vi "MeasAction.vi"(8 "error in (no error)":errorcluster caption="entrée d'erreur (pas d'erreur)", 9 "CurvePointIndex":i32, 10 "AllPointIndex":i32, 11 "InstrClassIn":refnum<class "LSCI332.lvclass"> caption="DNL_LabVIEW Object in") -> (0 "error out":errorcluster caption="sortie d'erreur", 2 "MeasDatOut":dbl[](array[numeric]), 3 "InstrClassOut":refnum<class "LSCI332.lvclass"> caption="DNL_LabVIEW Object out")   [LabVIEW 2019, in "LSCI332.lvclass"]
uses:
  LSCI332.lvclass
  C:/Programmes LabView/LabScanV1A/DevicesClass/BaseDevice/BaseDevice.lvclass
  LSCI332.lvclass/LSCI332.ctl
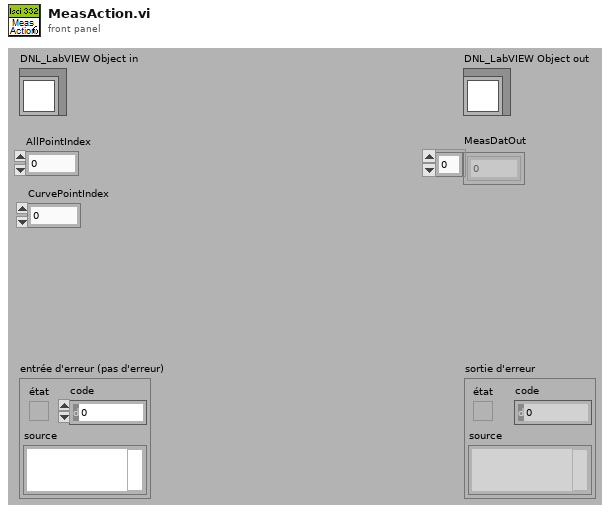
[diagram p1: front panel]
types:
  T1 = typedef "LSCI332.lvclass/LSCI332_Func.ctl" = enum16{"Read_InputA (K,S)", "Read_InputA&Heater (K,S,%,W)", "Read_InputB (K,S)", "Read_InputB&Heater (K,S,%,W)", "Read_Heater (%,W)", "Read_InputA&B(K,S,K,S)", "Read_InputA&B&Heater (K,S,K,S,%,W)", "Scan_Loop1(K,S)", "Scan_Loop2(K,S)"}
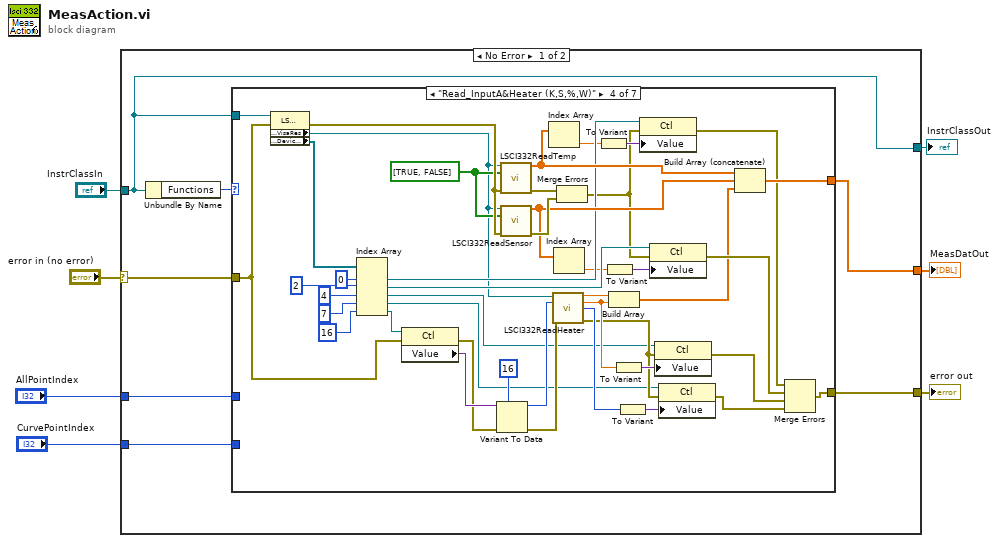
[diagram p0: block diagram]
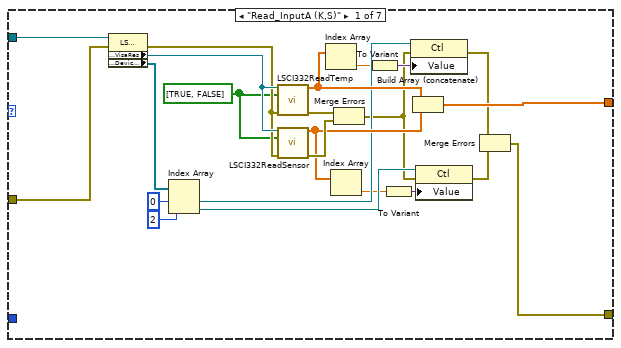
[diagram p2: hidden frame]
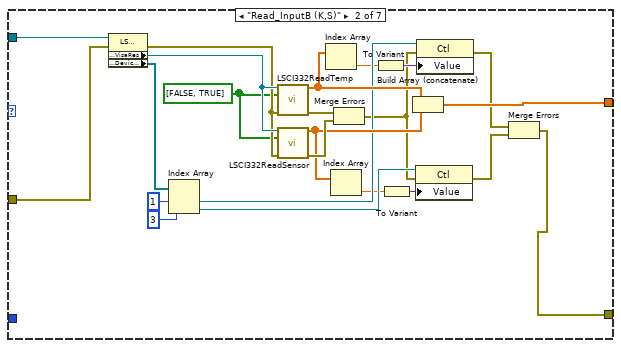
[diagram p3: hidden frame]
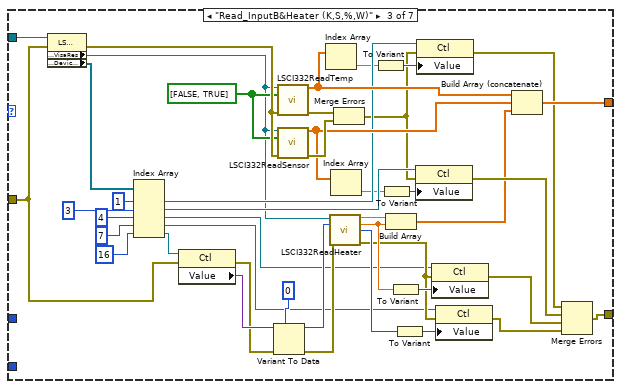
[diagram p4: hidden frame]
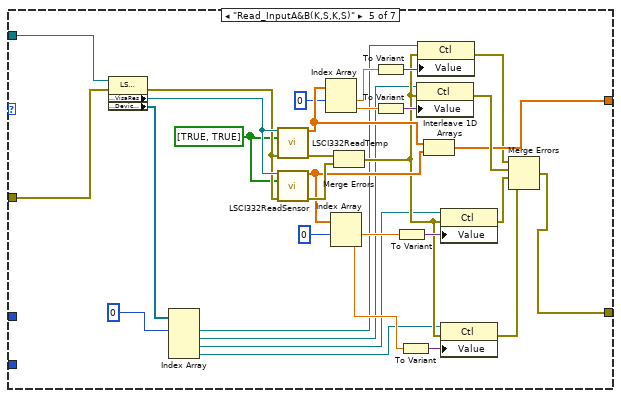
[diagram p5: hidden frame]
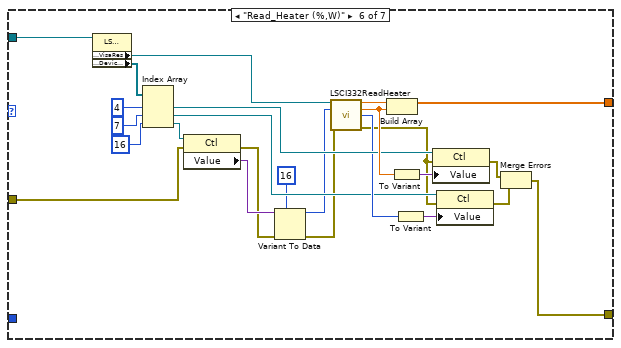
[diagram p6: hidden frame]
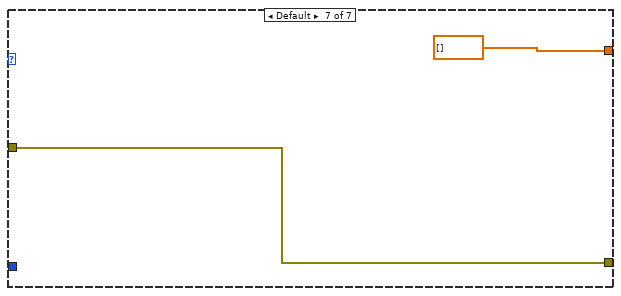
[diagram p7: hidden frame]
diagram:
  n1 = case shown="No Error" "error in (no error)" {
    selector: "error in (no error)" -> [w10 w206]
    tunnel: "InstrClassIn" -> [w8 w207]
    tunnel: [w8 w207] -> w5
    tunnel: "AllPointIndex" -> [w14 _]
    tunnel: [w13 w206] -> w3
    tunnel: [w12 _] -> w2
    tunnel: "CurvePointIndex" -> [w9 _]
    frame No Error {
      n2 = Unbundle By Name(w8) -> ("Functions"=w11:T1)
      n3 = case shown="\"Read_InputA&Heater (K,S,%,W)\"" w11 {
        tunnel: w14 -> [_ _ _ _ _ _ _]
        tunnel: [w17 w40 w85 w128 w165 w188 w204] -> w13
        tunnel: [w30 w53 w98 w141 w162 w202 dbl[] [] ("Outputs")] -> w12
        tunnel: w10 -> [w36 w59 w68 w111 w177 w183 w204]
        tunnel: w9 -> [_ _ _ _ _ _ _]
        tunnel: w8 -> [w37 w60 w103 w146 w178 w201 _]
        frame "Read_InputA (K,S)" {
          w33 = bool[] [TRUE, FALSE] ("Activées")
          n4 = property class="LSCI332.lvclass"(reference=w37, error in=w36) -> (error out=w34:errorcluster, "Accessor:VisaRes"=w35:refnum<visa-resource-name>, "Accessor:DeviceCtrl"=w29:refnum<vi>[])  [unwired: 1 out]
          n5 = Index Array(array=w29, index #1=0 ("index"), index #2=2 ("index")) -> (element #1=w26:refnum<vi>, element #2=w25:refnum<vi>)
          n6 = call <userlib>:"LSCI332ReadTemp.vi"("VISA Rsrc"=w35, "Activées"=w33, "error in"=w34) -> ("Données"=w28:dbl[], "error out"=w32:errorcluster)  [unwired: 11 in]
          n7 = call <userlib>:"LSCI332ReadSensor.vi"("VISA Rsrc"=w35, "Activées"=w33, "error in"=w34) -> ("Données"=w27:dbl[], "error out"=w31:errorcluster)  [unwired: 11 in]
          n8 = Index Array(array=w28) -> (element=w22:dbl)  [unwired: 1 in]
          n9 = Index Array(array=w27) -> (element=w24:dbl)  [unwired: 1 in]
          n10 = Merge Errors(w32, w31) -> (w20:errorcluster)
          n11 = To Variant(anything=w22) -> (Variant=w21:variant)
          n12 = To Variant(anything=w24) -> (Variant=w23:variant)
          n13 = property class="Ctl"(reference=w26, error in=w20, "Value"=w21) -> (error out=w19:errorcluster)  [unwired: 1 out]
          n14 = Build Array (concatenate)(w28, w27) -> (w30:dbl[])
          n15 = property class="Ctl"(reference=w25, error in=w20, "Value"=w23) -> (error out=w18:errorcluster)  [unwired: 1 out]
          n16 = Merge Errors(w19, w18) -> (w17:errorcluster)
        }
        frame "Read_InputB (K,S)" {
          w56 = bool[] [FALSE, TRUE] ("Activées")
          n17 = property class="LSCI332.lvclass"(reference=w60, error in=w59) -> (error out=w57:errorcluster, "Accessor:VisaRes"=w58:refnum<visa-resource-name>, "Accessor:DeviceCtrl"=w52:refnum<vi>[])  [unwired: 1 out]
          n18 = Index Array(array=w52, index #1=1 ("index"), index #2=3 ("index")) -> (element #1=w49:refnum<vi>, element #2=w48:refnum<vi>)
          n19 = call <userlib>:"LSCI332ReadTemp.vi"("VISA Rsrc"=w58, "Activées"=w56, "error in"=w57) -> ("Données"=w51:dbl[], "error out"=w55:errorcluster)  [unwired: 11 in]
          n20 = call <userlib>:"LSCI332ReadSensor.vi"("VISA Rsrc"=w58, "Activées"=w56, "error in"=w57) -> ("Données"=w50:dbl[], "error out"=w54:errorcluster)  [unwired: 11 in]
          n21 = Index Array(array=w51) -> (element=w45:dbl)  [unwired: 1 in]
          n22 = Index Array(array=w50) -> (element=w47:dbl)  [unwired: 1 in]
          n23 = Merge Errors(w55, w54) -> (w41:errorcluster)
          n24 = To Variant(anything=w45) -> (Variant=w44:variant)
          n25 = To Variant(anything=w47) -> (Variant=w46:variant)
          n26 = Build Array (concatenate)(w51, w50) -> (w53:dbl[])
          n27 = property class="Ctl"(reference=w48, error in=w41, "Value"=w46) -> (error out=w42:errorcluster)  [unwired: 1 out]
          n28 = property class="Ctl"(reference=w49, error in=w41, "Value"=w44) -> (error out=w43:errorcluster)  [unwired: 1 out]
          n29 = Merge Errors(w43, w42) -> (w40:errorcluster)
        }
        frame "Read_InputB&Heater (K,S,%,W)" {
          w101 = bool[] [FALSE, TRUE] ("Activées")
          n30 = property class="LSCI332.lvclass"(reference=w103, error in=w68) -> (error out=w102:errorcluster, "Accessor:VisaRes"=w65:refnum<visa-resource-name>, "Accessor:DeviceCtrl"=w97:refnum<vi>[])  [unwired: 1 out]
          n31 = Index Array(array=w97, index #1=1 ("index"), index #2=3 ("index"), index #3=4 ("index"), index #4=7 ("index"), index #5=16 ("index")) -> (element #1=w94:refnum<vi>, element #2=w93:refnum<vi>, element #3=w67:refnum<vi>, element #4=w66:refnum<vi>, element #5=w69:refnum<vi>)
          n32 = property class="Ctl"(reference=w69, error in=w68) -> (error out=w73:errorcluster, "Value"=w74:variant)  [unwired: 1 out]
          n33 = Variant To Data(error in=w73, type=u16 0 ("index"), Variant=w74) -> (data=w71:u16, error out=w70:errorcluster)
          n34 = call <userlib>:"LSCI332ReadTemp.vi"("VISA Rsrc"=w65, "Activées"=w101, "error in"=w102) -> ("Données"=w96:dbl[], "error out"=w100:errorcluster)  [unwired: 11 in]
          n35 = call <userlib>:"LSCI332ReadSensor.vi"("VISA Rsrc"=w65, "Activées"=w101, "error in"=w102) -> ("Données"=w95:dbl[], "error out"=w99:errorcluster)  [unwired: 11 in]
          n36 = Index Array(array=w96) -> (element=w90:dbl)  [unwired: 1 in]
          n37 = call <userlib>:"LSCI332ReadHeater.vi"("VISA Rsrc"=w65, "Résistance"=w71, "error in"=w70) -> ("Puissance(W)"=w80:dbl, "Puissance(%)"=w77:dbl, "Échelle"=w76:u16, "error out"=w75:errorcluster)  [unwired: 9 in]
          n38 = Index Array(array=w95) -> (element=w92:dbl)  [unwired: 1 in]
          n39 = Merge Errors(w100, w99) -> (w86:errorcluster)
          n40 = To Variant(anything=w90) -> (Variant=w89:variant)
          n41 = To Variant(anything=w92) -> (Variant=w91:variant)
          n42 = Build Array(w80, w77) -> (w64:dbl[])
          n43 = To Variant(anything=w77) -> (Variant=w79:variant)
          n44 = To Variant(anything=w76) -> (Variant=w78:variant)
          n45 = property class="Ctl"(reference=w93, error in=w86, "Value"=w91) -> (error out=w87:errorcluster)  [unwired: 1 out]
          n46 = property class="Ctl"(reference=w94, error in=w86, "Value"=w89) -> (error out=w88:errorcluster)  [unwired: 1 out]
          n47 = property class="Ctl"(reference=w67, error in=w75, "Value"=w79) -> (error out=w62:errorcluster)  [unwired: 1 out]
          n48 = property class="Ctl"(reference=w66, error in=w75, "Value"=w78) -> (error out=w63:errorcluster)  [unwired: 1 out]
          n49 = Build Array (concatenate)(w96, w95, w64) -> (w98:dbl[])
          n50 = Merge Errors(w88, w87, w62, w63) -> (w85:errorcluster)
        }
        frame "Read_InputA&Heater (K,S,%,W)" {
          w144 = bool[] [TRUE, FALSE] ("Activées")
          n51 = property class="LSCI332.lvclass"(reference=w146, error in=w111) -> (error out=w145:errorcluster, "Accessor:VisaRes"=w108:refnum<visa-resource-name>, "Accessor:DeviceCtrl"=w140:refnum<vi>[])  [unwired: 1 out]
          n52 = Index Array(array=w140, index #1=0 ("index"), index #2=2 ("index"), index #3=4 ("index"), index #4=7 ("index"), index #5=16 ("index")) -> (element #1=w137:refnum<vi>, element #2=w136:refnum<vi>, element #3=w110:refnum<vi>, element #4=w109:refnum<vi>, element #5=w112:refnum<vi>)
          n53 = property class="Ctl"(reference=w112, error in=w111) -> (error out=w116:errorcluster, "Value"=w117:variant)  [unwired: 1 out]
          n54 = Variant To Data(error in=w116, type=u16 16 ("index"), Variant=w117) -> (data=w114:u16, error out=w113:errorcluster)
          n55 = call <userlib>:"LSCI332ReadTemp.vi"("VISA Rsrc"=w108, "Activées"=w144, "error in"=w145) -> ("Données"=w139:dbl[], "error out"=w143:errorcluster)  [unwired: 11 in]
          n56 = call <userlib>:"LSCI332ReadSensor.vi"("VISA Rsrc"=w108, "Activées"=w144, "error in"=w145) -> ("Données"=w138:dbl[], "error out"=w142:errorcluster)  [unwired: 11 in]
          n57 = Index Array(array=w139) -> (element=w133:dbl)  [unwired: 1 in]
          n58 = call <userlib>:"LSCI332ReadHeater.vi"("VISA Rsrc"=w108, "Résistance"=w114, "error in"=w113) -> ("Puissance(W)"=w123:dbl, "Puissance(%)"=w120:dbl, "Échelle"=w119:u16, "error out"=w118:errorcluster)  [unwired: 9 in]
          n59 = Index Array(array=w138) -> (element=w135:dbl)  [unwired: 1 in]
          n60 = Merge Errors(w143, w142) -> (w129:errorcluster)
          n61 = To Variant(anything=w133) -> (Variant=w132:variant)
          n62 = To Variant(anything=w135) -> (Variant=w134:variant)
          n63 = Build Array(w123, w120) -> (w107:dbl[])
          n64 = To Variant(anything=w120) -> (Variant=w122:variant)
          n65 = To Variant(anything=w119) -> (Variant=w121:variant)
          n66 = property class="Ctl"(reference=w137, error in=w129, "Value"=w132) -> (error out=w131:errorcluster)  [unwired: 1 out]
          n67 = property class="Ctl"(reference=w136, error in=w129, "Value"=w134) -> (error out=w130:errorcluster)  [unwired: 1 out]
          n68 = property class="Ctl"(reference=w110, error in=w118, "Value"=w122) -> (error out=w105:errorcluster)  [unwired: 1 out]
          n69 = property class="Ctl"(reference=w109, error in=w118, "Value"=w121) -> (error out=w106:errorcluster)  [unwired: 1 out]
          n70 = Build Array (concatenate)(w139, w138, w107) -> (w141:dbl[])
          n71 = Merge Errors(w131, w130, w105, w106) -> (w128:errorcluster)
        }
        frame "Read_InputA&B(K,S,K,S)" {
          w174 = bool[] [TRUE, TRUE] ("Activées")
          n72 = property class="LSCI332.lvclass"(reference=w178, error in=w177) -> (error out=w175:errorcluster, "Accessor:VisaRes"=w176:refnum<visa-resource-name>, "Accessor:DeviceCtrl"=w171:refnum<vi>[])  [unwired: 1 out]
          n73 = Index Array(array=w171, index #1=0 ("index")) -> (element #1=w153:refnum<vi>, element #2=w152:refnum<vi>, element #3=w151:refnum<vi>, element #4=w150:refnum<vi>)  [unwired: 3 in]
          n74 = call <userlib>:"LSCI332ReadTemp.vi"("VISA Rsrc"=w176, "Activées"=w174, "error in"=w175) -> ("Données"=w164:dbl[], "error out"=w173:errorcluster)  [unwired: 11 in]
          n75 = call <userlib>:"LSCI332ReadSensor.vi"("VISA Rsrc"=w176, "Activées"=w174, "error in"=w175) -> ("Données"=w163:dbl[], "error out"=w172:errorcluster)  [unwired: 11 in]
          n76 = Index Array(array=w164, index #1=0 ("index")) -> (element #1=w157:dbl, element #2=w154:dbl)  [unwired: 1 in]
          n77 = Index Array(array=w163, index #1=0 ("index")) -> (element #1=w170:dbl, element #2=w158:dbl)  [unwired: 1 in]
          n78 = Merge Errors(w173, w172) -> (w160:errorcluster)
          n79 = To Variant(anything=w157) -> (Variant=w161:variant)
          n80 = To Variant(anything=w154) -> (Variant=w168:variant)
          n81 = To Variant(anything=w170) -> (Variant=w169:variant)
          n82 = To Variant(anything=w158) -> (Variant=w159:variant)
          n83 = property class="Ctl"(reference=w152, error in=w160, "Value"=w168) -> (error out=w167:errorcluster)  [unwired: 1 out]
          n84 = property class="Ctl"(reference=w153, error in=w160, "Value"=w161) -> (error out=w149:errorcluster)  [unwired: 1 out]
          n85 = Interleave 1D Arrays(w164, w163) -> (w162:dbl[])
          n86 = property class="Ctl"(reference=w151, error in=w160, "Value"=w169) -> (error out=w166:errorcluster)  [unwired: 1 out]
          n87 = property class="Ctl"(reference=w150, error in=w160, "Value"=w159) -> (error out=w148:errorcluster)  [unwired: 1 out]
          n88 = Merge Errors(w149, w167, w166, w148) -> (w165:errorcluster)
        }
        frame "Read_Heater (%,W)" {
          n89 = property class="LSCI332.lvclass"(reference=w201) -> ("Accessor:VisaRes"=w200:refnum<visa-resource-name>, "Accessor:DeviceCtrl"=w198:refnum<vi>[])  [unwired: 1 in, 2 out]
          n90 = Index Array(array=w198, index #1=4 ("index"), index #2=7 ("index"), index #3=16 ("index")) -> (element #1=w194:refnum<vi>, element #2=w192:refnum<vi>, element #3=w185:refnum<vi>)
          n91 = property class="Ctl"(reference=w185, error in=w183) -> (error out=w182:errorcluster, "Value"=w184:variant)  [unwired: 1 out]
          n92 = Variant To Data(error in=w182, type=u16 16 ("index"), Variant=w184) -> (data=w180:u16, error out=w179:errorcluster)
          n93 = call <userlib>:"LSCI332ReadHeater.vi"("VISA Rsrc"=w200, "Résistance"=w180, "error in"=w179) -> ("Puissance(W)"=w203:dbl, "Puissance(%)"=w196:dbl, "Échelle"=w193:u16, "error out"=w191:errorcluster)  [unwired: 9 in]
          n94 = Build Array(w203, w196) -> (w202:dbl[])
          n95 = To Variant(anything=w196) -> (Variant=w199:variant)
          n96 = To Variant(anything=w193) -> (Variant=w197:variant)
          n97 = property class="Ctl"(reference=w194, error in=w191, "Value"=w199) -> (error out=w190:errorcluster)  [unwired: 1 out]
          n98 = property class="Ctl"(reference=w192, error in=w191, "Value"=w197) -> (error out=w189:errorcluster)  [unwired: 1 out]
          n99 = Merge Errors(w190, w189) -> (w188:errorcluster)
        }
        frame Default {
        }
      }
    }
    frame Error {
    }
  }
  "error out" <- w3
  "InstrClassOut" <- w5
  "MeasDatOut" <- w2
